vi "dfd_Masking Filter Design for Super High Ratio Multirate Filter Design.vi"(5 "CIC order":i32, 6 "CIC factor":i32=5, 7 "CIC stage":i32=3, 8 "error in (no error)":errorcluster, 9 "ripple specs":T1={"passband"=0.03624968728875148, "stopband"=0.001, "dB/linear? (T: dB)"=FALSE}, 10 "fstop":dbl=0.25, 11 "fpass":dbl=0.06818181818181818) -> (0 "error out":errorcluster, 3 "filter out":T2={"mSRate_Fs"=1.0, "mSRate_Version"="1.0", "mSRate_Comments"="", "mSRate_OrgCoef"={"type"=enum."Undefined", "gain"=1.0, "coef a (k)"=[], "coef b (v)"=[]}, "mSRate_CurCoef"={"type"=enum."Undefined", "gain"=1.0, "coef a (k)"=[], "coef b (v)"=[]}, "mSRate_Quantized?"=FALSE, "mSRate_QCoef"={"type"=enum."Undefined", "gain"=1.0, "coef a (k)"=[], "coef b (v)"=[]}, "mSRate_QSettings"=[], "mSRate_Order"=0, "mSRate_Scaling"={"mSRate_ScaleByPowerOf2?"=FALSE, "mSRate_ScaleType"=enum."No Norm"}} {"mSRate_QSettings"."source" items=["Coef a/k"=0, "Coef b/v"=7, "Input"=1, "Output"=2, "Multiplicand"=3, "Product"=4, "Sum"=5, "Delay"=6, "Gain"=8]})   [LabVIEW 2017, in "NI_DigFilter_Process.lvlib"]
uses:
  <vilib>/addons/Digital Filter Design/NI_DigFilter_Process.lvlib
  <vilib>/addons/Digital Filter Design/_Objects.llb/DFD Filter Obj.ctl
  <vilib>/addons/Digital Filter Design/_Objects.llb/DFD Filter Coef.ctl
  <vilib>/addons/Digital Filter Design/_Objects.llb/DFD Filter Structure Type Selector.ctl
  <vilib>/addons/Digital Filter Design/_Objects.llb/dfd_Internal Quantization Settings.ctl
  <vilib>/addons/Digital Filter Design/_Objects.llb/dfd_Internal Quantization Srcs.ctl
  <vilib>/addons/Digital Filter Design/_Objects.llb/DFD Coef Norm Type.ctl
  <vilib>/addons/Digital Filter Design/_Objects.llb/DFD Filter Ripple Specification (Design).ctl
  <vilib>/addons/Digital Filter Design/_REMEZ.llb/remez_fir filter type.ctl
  <vilib>/addons/Digital Filter Design/_Objects.llb/DFD Filter Frequence Specification (Design).ctl
  <vilib>/addons/Digital Filter Design/NI_DigFilterLicensed.lvlib
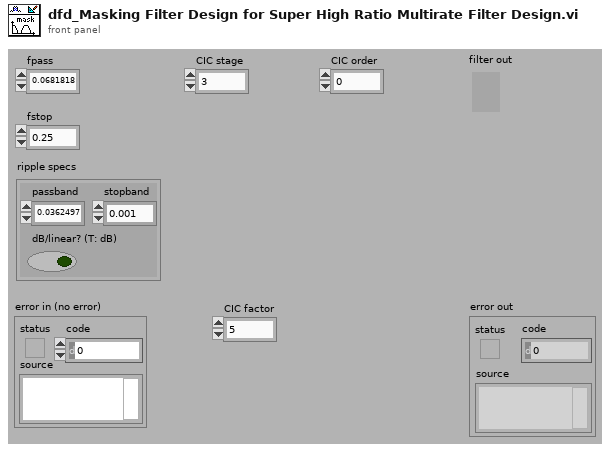
[diagram p1: front panel]
types:
  T1 = typedef "NI_DigFilterLicensed.lvlib/DFD Filter Ripple Specification (Design).ctl" = cluster{"passband":dbl, "stopband":dbl, "dB/linear? (T: dB)":bool}
  T2 = typedef "NI_DigFilterLicensed.lvlib/DFD Filter Obj.ctl" = cluster{"mSRate_Fs":dbl, "mSRate_Version":string, "mSRate_Comments":string, "mSRate_OrgCoef":T3, "mSRate_CurCoef":T3, "mSRate_Quantized?":bool, "mSRate_QCoef":T3, "mSRate_QSettings":T5[], "mSRate_Order":i32, "mSRate_Scaling":cluster{"mSRate_ScaleByPowerOf2?":bool, "mSRate_ScaleType":T7}}
  T3 = typedef "NI_DigFilterLicensed.lvlib/DFD Filter Coef.ctl" = cluster{"type":T4, "gain":dbl, "coef a (k)":dbl[], "coef b (v)":dbl[]}
  T4 = typedef "NI_DigFilterLicensed.lvlib/DFD Filter Structure Type Selector.ctl" = enum16{"Undefined", "FIR Direct Form", "FIR Direct Form Transposed", "FIR Symmetric", "FIR Antisymmetric", "IIR Direct Form I", "IIR Direct Form I Transposed", "IIR Direct Form II", "IIR Direct Form II Transposed", "IIR Cascaded Second Order Sections Form I", "IIR Cascaded Second Order Sections Form I Transposed", "IIR Cascaded Second Order Sections Form II", "IIR Cascaded Second Order Sections Form II Transposed", "Lattice Allpass (basic sections)", "Lattice Allpass (one multiplier sections)", "Lattice Allpass (normalized sections)", "Lattice AR (basic sections)", "Lattice AR (one multiplier sections)", "Lattice AR (normalized sections)", "Lattice MA (minimum phase)", "Lattice MA (maximum phase)", "Lattice ARMA (basic sections)", "Lattice ARMA (one multiplier sections)", "Lattice ARMA (normalized sections)"}
  T5 = typedef "NI_DigFilterLicensed.lvlib/dfd_Internal Quantization Settings.ctl" = cluster{"source":T6, "wl":i16, "iwl":i16, "overflow mode":enum16{"Saturation", "Wrap"}, "rounding mode":enum16{"Nearest", "Truncation"}, "signed?":bool}
  T6 = typedef "NI_DigFilterLicensed.lvlib/dfd_Internal Quantization Srcs.ctl" = u16
  T7 = typedef "NI_DigFilterLicensed.lvlib/DFD Coef Norm Type.ctl" = enum16{"No Norm", "Time Domain 1-Norm", "Time Domain 2-Norm", "Time Domain Inf-Norm"}
  T8 = typedef "NI_DigFilterLicensed.lvlib/DFD Filter Frequence Specification (Design).ctl" = cluster{"fpass 1":dbl, "fstop 1":dbl, "fpass 2 ":dbl, "fstop 2":dbl}
  T9 = typedef "NI_DigFilterLicensed.lvlib/remez_fir filter type.ctl" = enum32{"Symmetric", "Antisymmetric", "Differentiator", "Hilbert", "Minimum Phase", "Maximum Phase"}
  T10 = enum16{"Lowpass", "Highpass", "Bandpass", "Bandstop"}
  T11 = typedef "NI_DigFilterLicensed.lvlib/DFD Adv Band Spec.ctl" = cluster{"band specification":cluster{"freq":dbl, "amplitude":dbl, "weight":dbl}[], "ripple constraint":dbl}
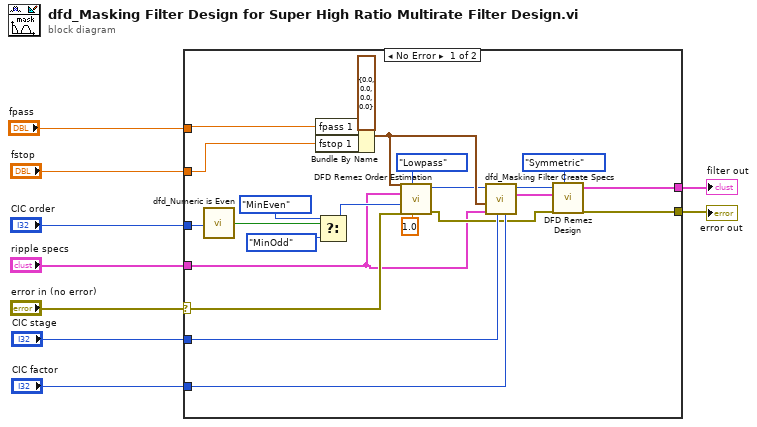
[diagram p0: block diagram]
diagram:
  n1 = case shown="No Error" "error in (no error)" {
    selector: "error in (no error)" -> [w28 w32]
    tunnel: [w26 w32] -> w9
    tunnel: [w27 _] -> w8
    tunnel: "CIC stage" -> [w13 _]
    tunnel: "fstop" -> [w18 _]
    tunnel: "fpass" -> [w19 _]
    tunnel: "CIC factor" -> [w12 _]
    tunnel: "CIC order" -> [w25 _]
    tunnel: "ripple specs" -> [w10 _]
    frame No Error {
      n2 = call <vilib>:"dfd_Numeric is Even.vi"("N"=w25) -> ("even ?"=w23:bool)
      n3 = Bundle By Name(cluster=T8 {"fpass 1"=0.0, "fstop 1"=0.0, "fpass 2 "=0.0, "fstop 2"=0.0} ("Shaping freq specs [Hz]"), "fpass 1"=w19, "fstop 1"=w18) -> (w17:T8)
      n4 = Select(t=enum16{"MinNum", "MinEven", "MinOdd"}."MinEven" ("order option"), s=w23, f=enum16{"MinNum", "MinEven", "MinOdd"}."MinOdd" ("order option")) -> (s? t:f=w21:enum16{"MinNum", "MinEven", "MinOdd"})
      n5 = call <vilib>:"DFD Remez Order Estimation.vi"("fs [Hz]"=1.0, "filter type"=T10."Lowpass", "error in (no error)"=w28, "order option"=w21, "ripple specs"=w10, "freq specs [Hz]"=w17) -> ("error out"=w11:errorcluster, "estimated order"=w16:i32)  [unwired: 4 out]
      n6 = call <vilib>:"dfd_Masking Filter Create Specs.vi"("CIC factor"=w12, "CIC stage"=w13, "ripple specs"=w10, "masking freq specs [Hz]"=w17, "masking order"=w16) -> ("Masking band parameters"=w14:T11[], "dup masking order"=w15:i32)  [unwired: 1 in, 4 out]
      n7 = call <vilib>:"DFD Remez Design.vi"("filter type"=remez_fir_filter_type."Symmetric", "error in (no error)"=w11, "band specs"=w14, "order"=w15) -> ("error out"=w26:errorcluster, "filter out"=w27:T2)  [unwired: 3 in, 3 out]
    }
    frame Error {
    }
  }
  "error out" <- w9
  "filter out" <- w8
